vi "Joystick and Camera.vi"() -> ()   [LabVIEW 2021]
uses:
  Classes/Controller/Camera/Machine Vision.ctl
  Classes/Controller/Camera/Image processing.ctl
  Classes/Controller/Camera/Camera settings.ctl
  <vilib>/vision/Pattern Matching.llb/IMAQ GM Match Report.ctl
  <vilib>/vision/Measure.llb/Edge New.ctl
  Classes/Controller/I-O/I-O.lvclass
  Classes/Controller/Camera/Camera.lvclass
  Classes/Controller/Controller.lvclass
  Classes/Controller/Motion/A3200/A3200.lvclass
  Classes/Controller/Motion/Motion.lvclass
  Test VIs/Test VIs.lvclass
panel:
  in  "Cluster":T1={"Bayer"={"Algorithm"=0, "Gain R"=1.0, "Gain B"=1.0, "Gain G"=1.0, "Pattern"=5}, "Acquisition Control"={"Trigger Selector"=0, "Acquisition Frame Rate"=20.0, "Exposure Time"=100.0, "Acquisition Frame Rate Target"=20.0}, "Analog Control"={"Black Level"=0.0, "Gain Selector"=10, "Gain"=1.0}} {"Analog Control"."Gain" min=1.0 max=15.0; "Analog Control"."Gain Selector" items=["Analog All"=10, "Digital All"=20]; "Analog Control"."Black Level" min=0.0 max=255.9375; "Acquisition Control"."Acquisition Frame Rate Target" min=0.001 max=150000000.0; "Acquisition Control"."Exposure Time" min=27.793333333333333 max=1048539.7933333333; "Acquisition Control"."Acquisition Frame Rate" min=0.9536888685435264 max=30.757874015748033; "Acquisition Control"."Trigger Selector" items=["Frame Start"=3, "Exposure Start"=10]; "Bayer"."Pattern" items=["Use hardware value"=5, "None"=0, "GB"=1, "GR"=2, "BG"=3, "RG"=4]; "Bayer"."Gain G" min=0.0 max=3.999; "Bayer"."Gain B" min=0.0 max=3.999; "Bayer"."Gain R" min=0.0 max=3.999; "Bayer"."Algorithm" items=["Bilinear", "VNG"]}
  out "Used Edges (Adv. Straight Edge 1)":cluster{"Edge Information":T2[]}[](array[cluster]) {"Edge Information"."Distance (Real-World)" format="%.2f"; "Edge Information"."Location (Real-World)"."Y" format="%.2g"; "Edge Information"."Location (Real-World)"."X" format="%.2f"; "Edge Information"."Noise" format="%.2f"; "Edge Information"."Location (Pixel)"."Y" format="%.2g"; "Edge Information"."Location (Pixel)"."X" format="%.2f"; "Edge Information"."Strength" format="%.2f"; "Edge Information"."Distance (Pixel)" format="%.2f"}
  out "pattern matching":T3 {"Correlation Score" format="%.2f"; "Target Template Curve Score" format="%.2f"; "Template Target Curve Score" format="%.2f"; "Bounding Box"."y" format="%.2f"; "Bounding Box"."x" format="%.2f"; "Position"."y" format="%.2f"; "Position"."x" format="%.2f"; "Score" format="%.2f"; "Scale" format="%.2f"; "Angle" format="%.2f"; "Occlusion %" format="%.2f"}
  out "Match?":bool
  out "Current position spiral":dbl[](array[numeric])
  in  "Z high":dbl=12.5
  in  "XY high":dbl=50.0
  in  "Z low":dbl=0.05
  in  "XY low":dbl=0.1
  out "Current Z High Speed":dbl
  out "Current XY High Speed":dbl
  out "current Z low speed":dbl
  out "current XY speed":dbl
  out "High Speed":bool
  out "Z":bool
  out "Y":bool
  out "X":bool
  out "Low Speed":bool
  out "Global Report":T4 {"Mean Value" format="%.2f"; "%" format="%.2f"; "Area (calibrated)" format="%.2f"; "Maximal Value" format="%.2f"; "Minimal Value" format="%.2f"; "Standard Variation" format="%.2f"}
  in  "MoveFour":dbl[][](array[numeric])=[[1280.0, 960.0], [-2560.0, 0.0], [0.0, -1920.0], [2560.0, 0.0], [-1280.0, 960.0]]
  in  "Check four images":bool
  in  "Go TL fid":bool
  in  "Find fiducial":bool
  in  "Loop count":dbl=1.0
  in  "X, Y pixel stride":dbl[](array[numeric])=[1520.0, 2160.0]
  in  "Draw spiral":bool
  out "Move by":dbl[](array[numeric])
  in  "Find in Image":bool
  in  "Screen Grab":bool
  in  "Focus step size":dbl format="%#_13g"
  in  "number of focus steps":i32
  out "Radius (Real-World)":dbl
  out "error out":errorcluster
  in  "Find fiducial center":bool
  out "maximum is best focus":dbl
  in  "Focus":bool
  in  "Override presets":bool
  in  "Camera settings":T5={"Gamma"=1.6, "Gain"=0, "Sharpness"=0, "Contrast"=0.0, "Exposure"=0.0078125} {"Exposure" min=0.000244140625 max=0.5 scale=0.0002..0.5; "Contrast" min=0.0 max=1.0 scale=0.0..1.0; "Sharpness" min=0 max=2 step=1 scale=0.0..2.0; "Gain" min=0 max=100 step=1 scale=0.0..100.0; "Gamma" min=0.01 max=10.0 scale=0.01..10.0}
  in  "Image processing":T6={"Brightness"=128.0, "Contrast"=45.0, "Gamma"=1.0471123} {"Brightness" scale=0.0..400.0; "Contrast" scale=0.0..90.0; "Gamma" scale=0.005..5.0}
  out "XYZTheta Out":dbl[](array[numeric])
  in  "Machine Vision":T7
  in  "Move 10cm Right":bool
  in  "Move 10cm Backward":bool
  in  "Move 10cm Forward":bool
  in  "Move 10cm Left":bool
  in  "Record Measurement":bool=TRUE
  in  "Dismount Silicon Tray":bool
  in  "Secure Silicon Tray":bool
  in  "Z Go":bool
  in  "Position":dbl
  in  "XYZTheta":dbl[](array[numeric])
  in  "Go":bool
  in  "Joystick":bool
  out "Sum":dbl[](array[numeric]) format="%#.6g"
  out "Gantry":dbl[](array[numeric]) format="%#.6g"
  in  "Stop":bool
  out "Image":T8(plugin-control)
  out "Camera":dbl[](array[numeric])
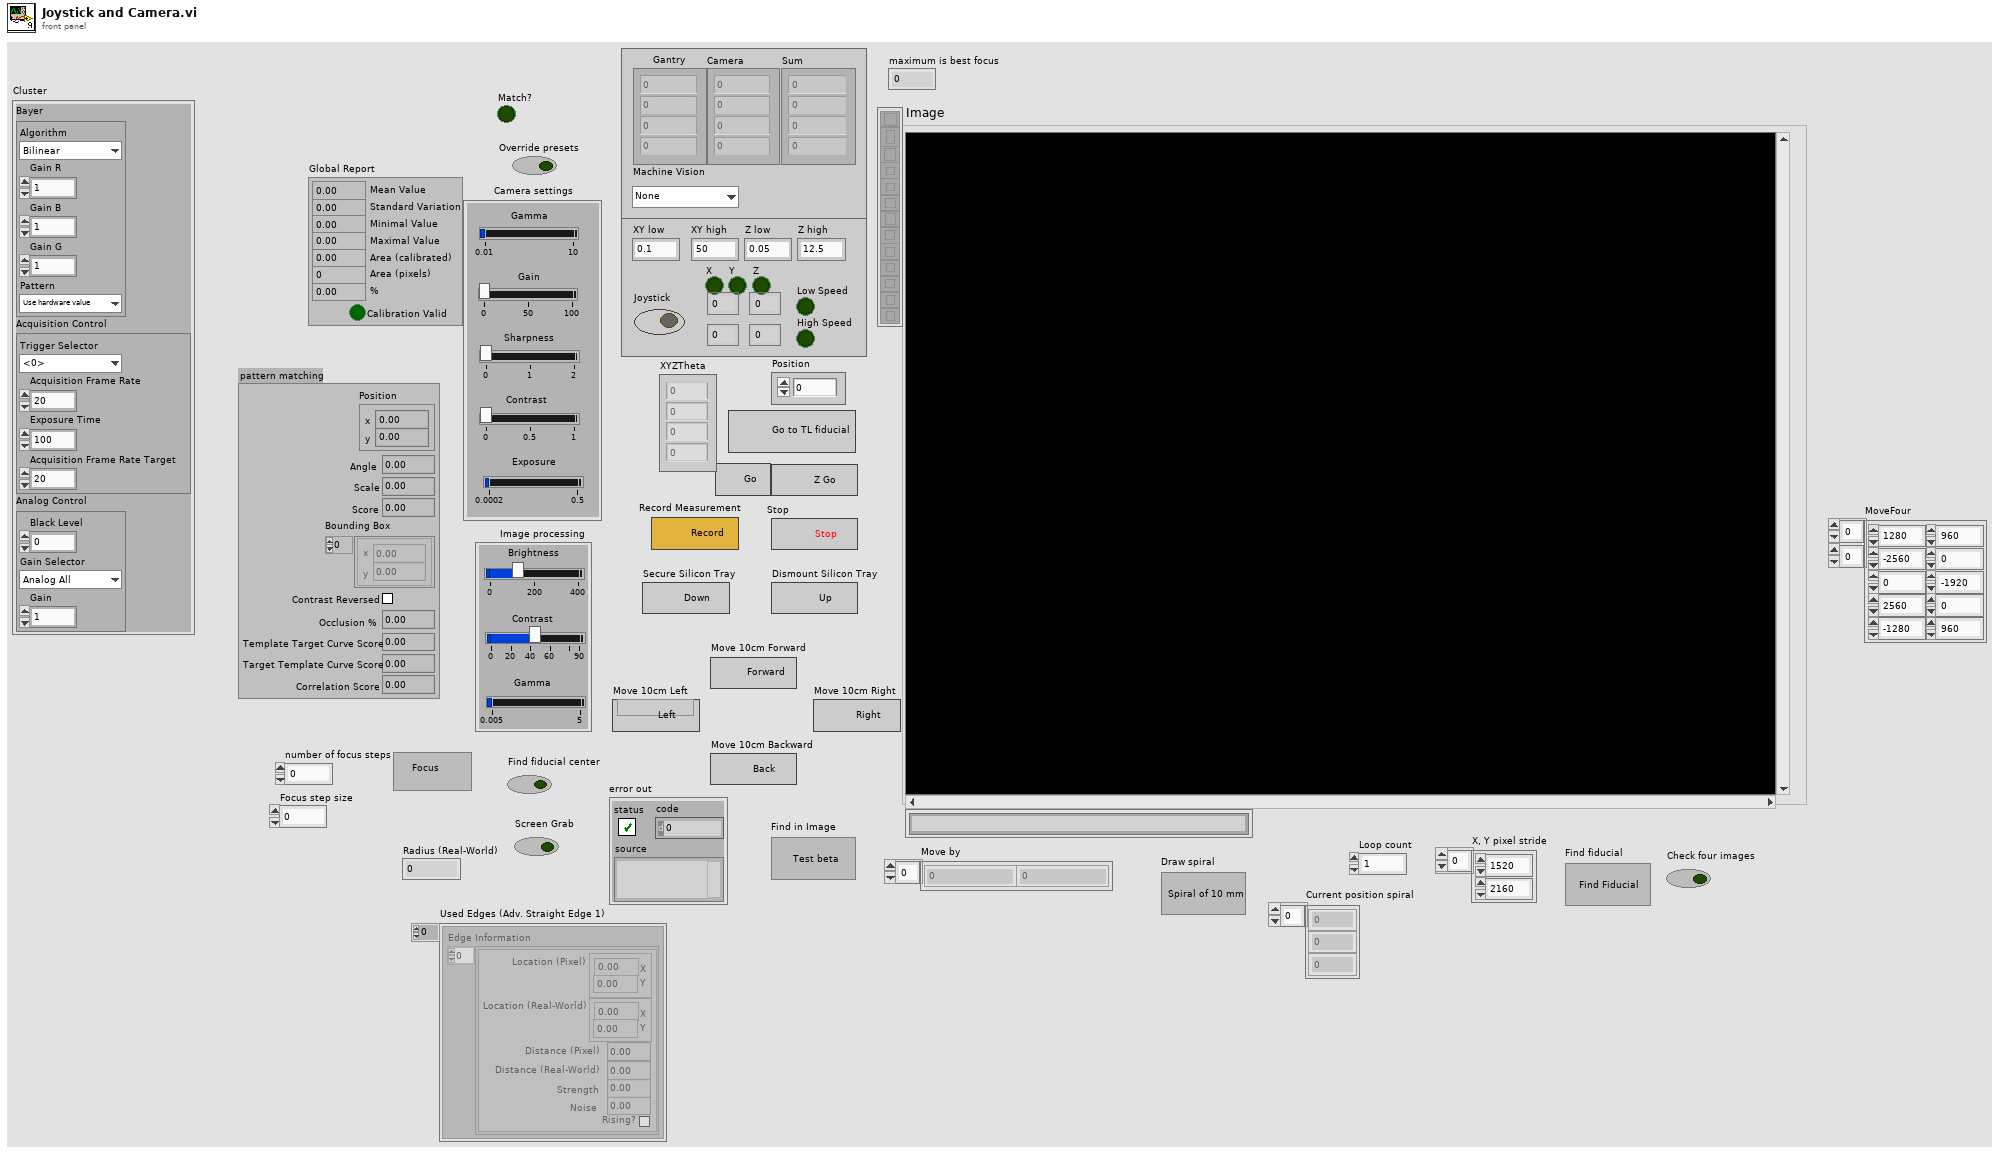
[diagram p1: front panel]
types:
  T1 = cluster{"Bayer":cluster{"Algorithm":u32, "Gain R":dbl, "Gain B":dbl, "Gain G":dbl, "Pattern":u32}, "Acquisition Control":cluster{"Trigger Selector":u32, "Acquisition Frame Rate":dbl, "Exposure Time":dbl, "Acquisition Frame Rate Target":dbl}, "Analog Control":cluster{"Black Level":dbl, "Gain Selector":u32, "Gain":dbl}}
  T2 = typedef "Edge New.ctl" = cluster{"Location (Pixel)":cluster{"X":sgl, "Y":sgl}, "Location (Real-World)":cluster{"X":sgl, "Y":sgl}, "Distance (Pixel)":dbl, "Distance (Real-World)":dbl, "Strength":dbl, "Noise":dbl, "Rising?":bool}
  T3 = typedef "IMAQ GM Match Report.ctl" = cluster{"Position":cluster{"x":sgl, "y":sgl}, "Angle":sgl, "Scale":sgl, "Score":sgl, "Bounding Box":cluster{"x":sgl, "y":sgl}[], "Contrast Reversed":bool, "Occlusion %":sgl, "Template Target Curve Score":sgl, "Target Template Curve Score":sgl, "Correlation Score":sgl}
  T4 = cluster{"Mean Value":sgl, "Standard Variation":sgl, "Minimal Value":sgl, "Maximal Value":sgl, "Area (calibrated)":sgl, "Area (pixels)":u32, "%":sgl, "Calibration Valid":bool}
  T5 = typedef "Camera.lvclass/Camera settings.ctl" = cluster{"Gamma":dbl, "Gain":i64, "Sharpness":i64, "Contrast":dbl, "Exposure":dbl}
  T6 = typedef "Camera.lvclass/Image processing.ctl" = cluster{"Brightness":sgl, "Contrast":sgl, "Gamma":sgl}
  T7 = typedef "Camera.lvclass/Machine Vision.ctl" = enum16{"None", "Assembly Tray Circle", "Assembly Tray Fiducial", "Partial Hexaboard", "sensor edge init", "HB edge init", "sensor edge pos1", "sensor edge pos2", "HB edge pos1", "HB edge pos2", "Sensor CH1-2", "HB CH1", "HB CH2", "V3 Sensor Circle", "Hexaboard Circle", "sensor CH1 check", "HB CH1 check ", "sensor ID"}
  T8 = typedef "IMAQ Image.ctl" = refnum<image>
  T9 = enum16{"open", "replace", "create", "open or create", "replace or create", "replace or create with confirmation"}
  T10 = typedef "Controller.lvclass/Controllers.ctl" = cluster{"I-O.lvclass":refnum<class "I-O.lvclass">, "Gantry":refnum<k24>, "Dispenser":refnum<visa-resource-name>}
  T11 = cluster{"Average Strength":dbl, "Radius (Real-World)":dbl, "Match found?":bool, "initial angle":sgl, "Global Report":cluster{"Mean Value":sgl, "Standard Variation":sgl, "Minimal Value":sgl, "Maximal Value":sgl, "Area (calibrated)":sgl, "Area (pixels)":u32, "%":sgl, "Calibration Valid":bool}}
  T12 = typedef "I-O.lvclass/Pin Map.ctl" = cluster{"Region Valves":i32[], "Extra Valves":dbl[][][], "Tool Primary Valve":i32, "Tool Secondary Valve":i32, "Region Sensors":i32[], "Extra Sensors":dbl[][][], "Tool Primary Sensor":dbl, "Tool Secondary Sensor":dbl, "Compression Sensor":dbl, "5V":i32, "Dispenser Sensor":dbl, "Light Curtain":i32}
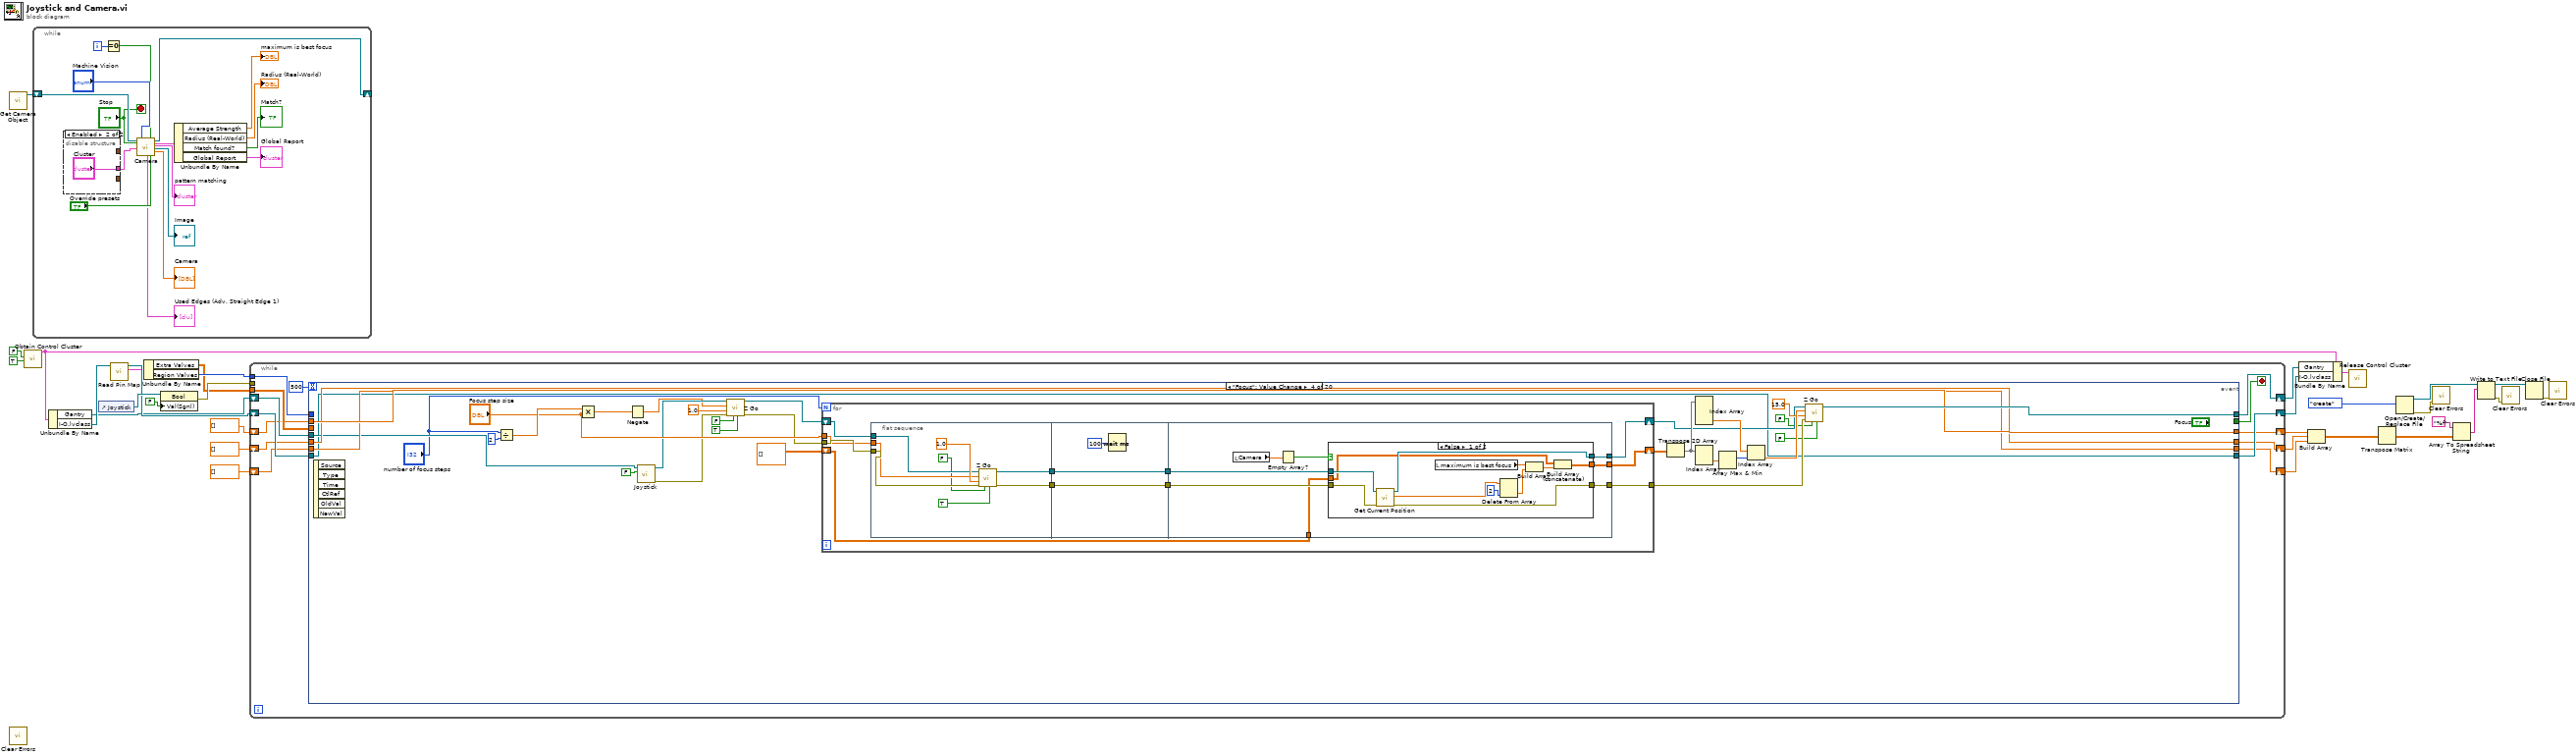
[diagram p0: block diagram]
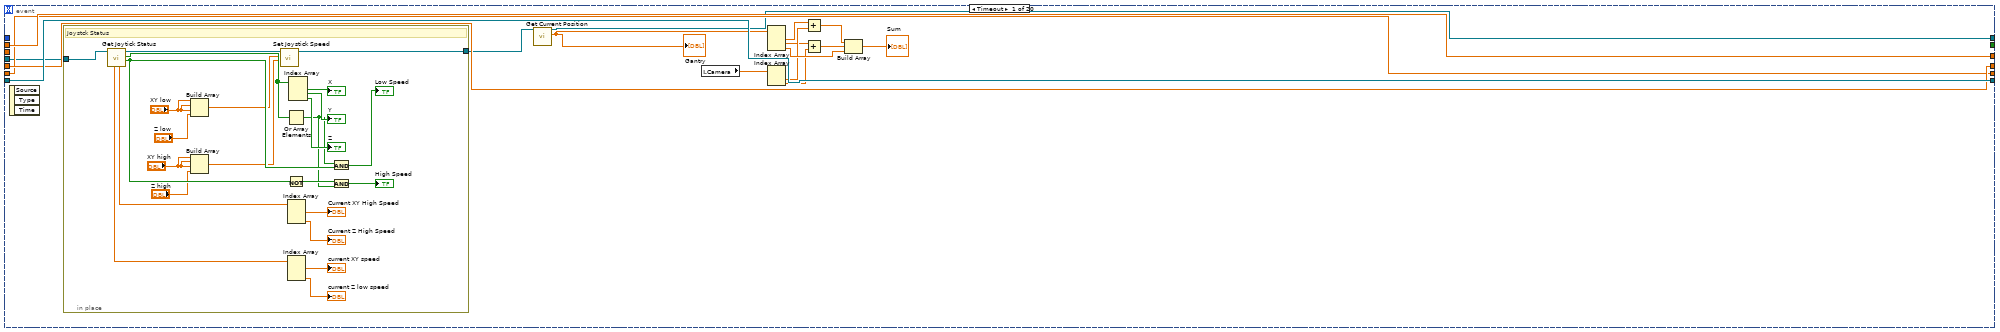
[diagram p2: hidden frame]
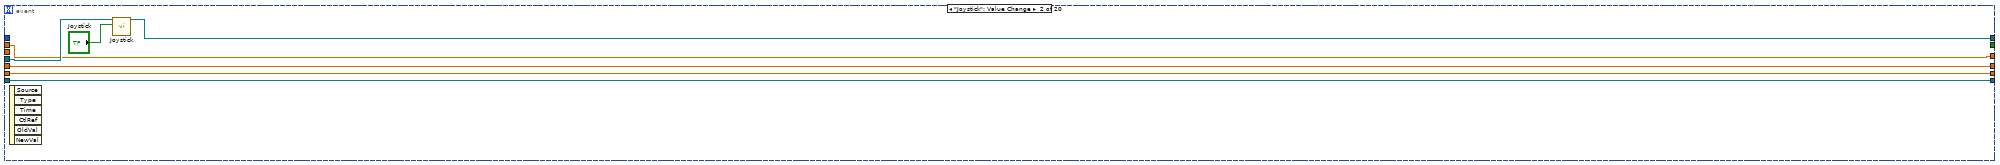
[diagram p3: hidden frame]
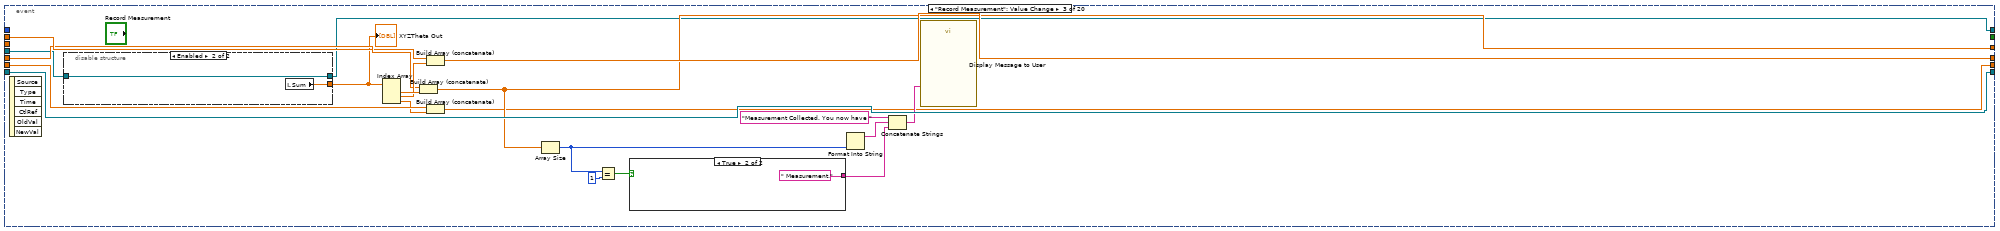
[diagram p4: hidden frame]
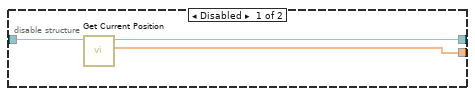
[diagram p5: hidden frame]
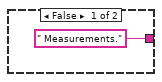
[diagram p6: hidden frame]
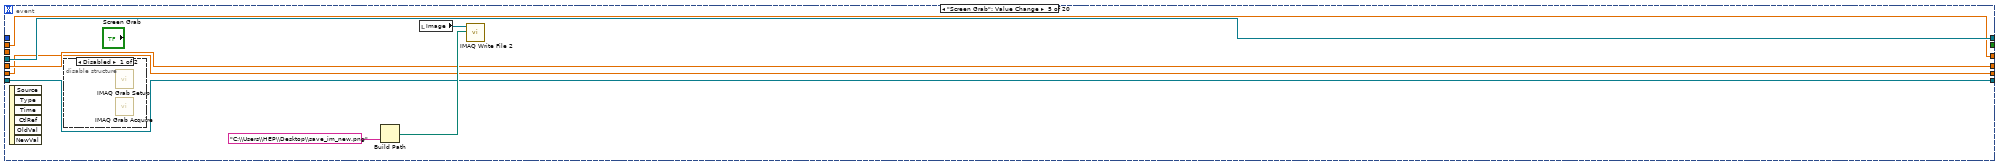
[diagram p8: hidden frame]
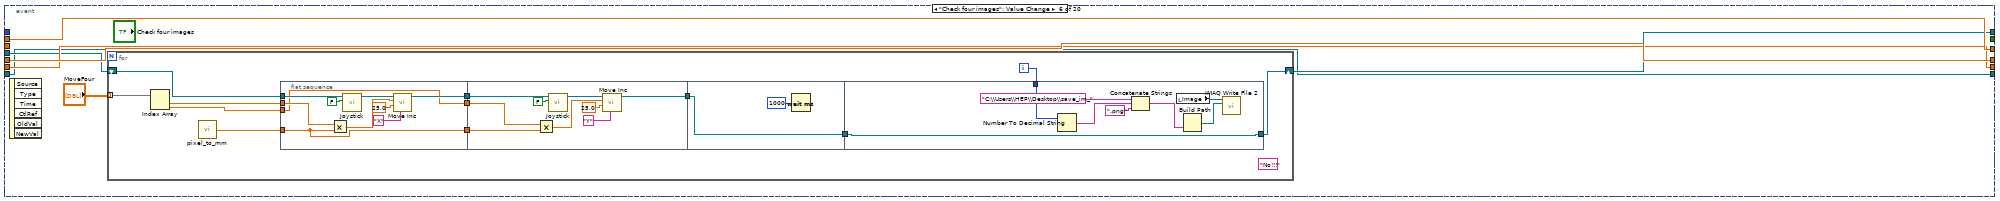
[diagram p10: hidden frame]
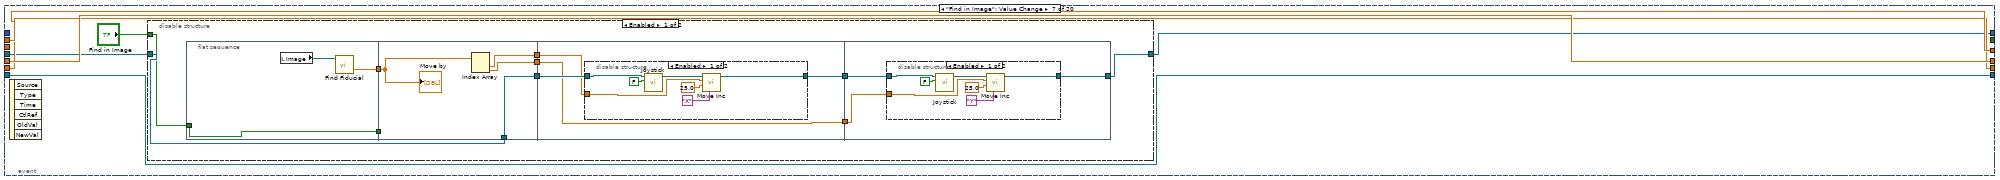
[diagram p11: hidden frame]
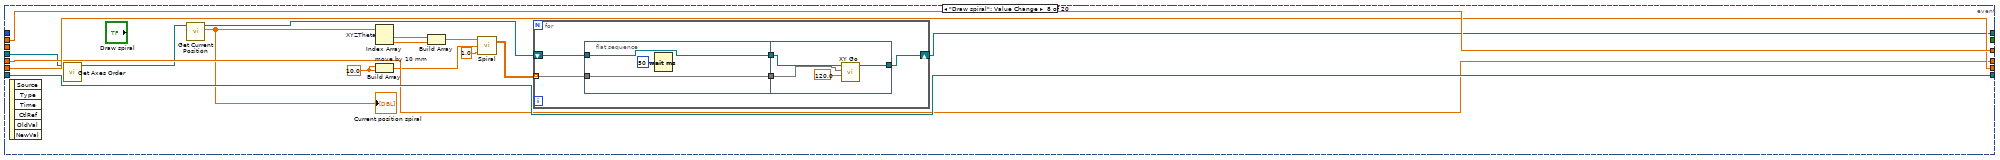
[diagram p15: hidden frame]
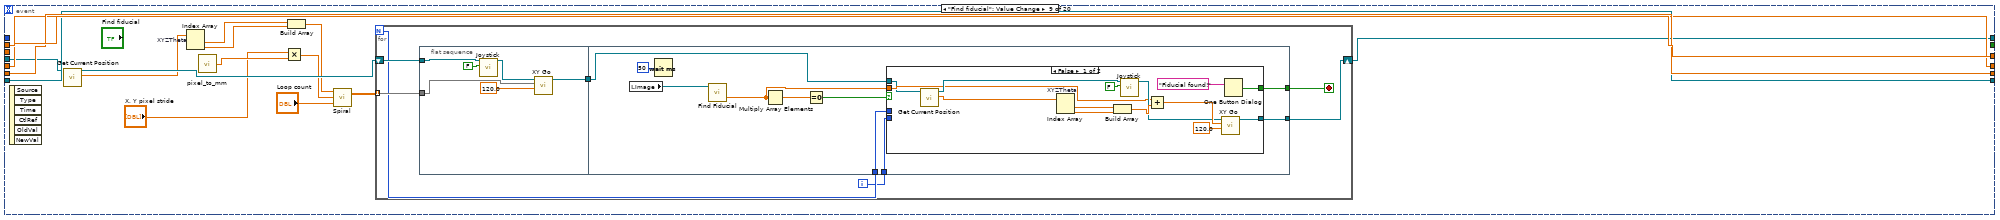
[diagram p16: hidden frame]
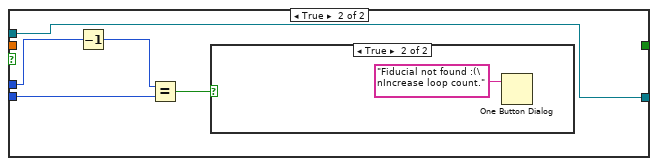
[diagram p17: hidden frame]
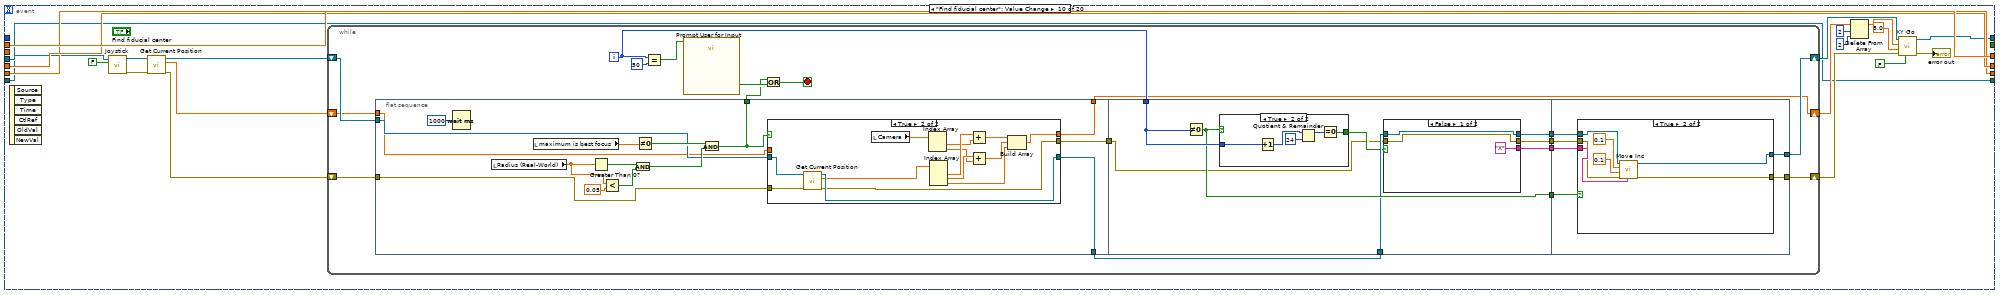
[diagram p19: hidden frame]
diagram:
  n1 = call "Get Camera Object.vi"() -> ("Camera out"=w27:refnum<class "Camera.lvclass">)  [unwired: 10 in, 1 out]
  n2 = call <vilib>:"Clear Errors.vi"() -> ()  [unwired: 6 in, 2 out]
  n3 = call "Obtain Control Cluster.vi"("I/O"=TRUE, "Dispense"=FALSE) -> ("Control Out"=w5:T10)  [unwired: 8 in, 1 out]
  n4 = while {
    shift-right: [w48] -> _
    shift-left: w27 -> [w49]
    i -> [w43]
    stop <- "Stop" stop-if-true
    n5 = disable-structure shown="Enabled" {
      disable-tunnel: ["Image processing" _] -> _
      disable-tunnel: ["Camera settings" _] -> _
      disable-tunnel: [_ "Cluster"] -> w33
      frame Disabled {
      }
      frame Enabled {
      }
    }
    n6 = Equal To 0?(x=w43) -> (x = 0?=w42:bool)
    n7 = call "Camera.vi"("Camera in"=w49, "Stop"="Stop", "Cluster"=w33, "Machine Vision"="Machine Vision", "Loop 0"=w42, "Override presets"="Override presets") -> ("Used Edges (Adv. Straight Edge 1)"=→"Used Edges (Adv. Straight Edge 1)":cluster{"Edge Information":T2[]}[], "Camera out"=w48:refnum<class "Camera.lvclass">, "output cluster"=w41:T11, "pattern matching"=→"pattern matching":T3, "Image"=→"Image":T8, "Camera"=→"Camera":dbl[])  [unwired: 6 in, 2 out]
    n8 = Unbundle By Name(w41) -> ("Average Strength"=→"maximum is best focus":dbl, "Radius (Real-World)"=→"Radius (Real-World)":dbl, "Match found?"=→"Match?":bool, "Global Report"=→"Global Report":T4)
  }
  n9 = Unbundle By Name(w5) -> ("Gantry"=w4:refnum<k24>, "I-O.lvclass"=w26:refnum<class "I-O.lvclass">)
  n10 = control-ref of="Joystick"() -> (w31:refnum<vi>)
  n11 = call-dynamic "Read Pin Map.vi"("I-O in"=w26) -> ("Pin Map 2"=w24:T12, "I-O out"=w25:refnum<class "I-O.lvclass">)  [unwired: 8 in, 1 out]
  n12 = Unbundle By Name(w24) -> ("Extra Valves"=w22:dbl[][][], "Region Valves"=w23:i32[])
  n13 = property class="Bool"(reference=w31, "Val(Sgnl)"=FALSE ("Value (Signaling)")) -> (error out=w30:errorcluster)  [unwired: 1 in, 1 out]
  n14 = while {
    shift-right: [w53] -> w8
    shift-left: w4 -> [w64]
    tunnel: w30 -> [_]
    shift-right: [w62] -> w7
    shift-left: w25 -> [w63]
    tunnel: w23 -> [w61]
    tunnel: w22 -> [w60]
    shift-right: [w55] -> w10
    shift-left: dbl[] [] -> [w59]
    shift-right: [w57] -> w11
    shift-left: dbl[] [] -> [w58]
    shift-right: [w54] -> w12
    shift-left: dbl[] [] -> [w56]
    stop <- w65 stop-if-true
    n15 = event shown="[3] \"Focus\": Value Change" {
      selector: _ -> [_ _ _ _ _ _ _ _ _ _ _ _ _ _ _ _ _ _ _ _]
      dyn-events: _ -> [_ _ _ _ _ _ _ _ _ _ _ _ _ _ _ _ _ _ _ _]
      timeout: 500 -> [_ _ _ _ _ _ _ _ _ _ _ _ _ _ _ _ _ _ _ _]
      tunnel: [_ _ _ _ _ _ _ _ _ _ _ _ _ _ _ _ _ _ _ TRUE] -> w65
      tunnel: w64 -> [w68 w114 w117 w159 w223 w229 w276 w323 w350 w426 w545 w556 w567 w578 w580 w590 w608 w627 w633 w670]
      tunnel: w63 -> [w83 w112 w134 w143 w222 w227 w280 w334 w363 w409 w540 w552 w564 w575 w587 w599 w605 w624 w637 w668]
      tunnel: [w83 w112 w134 w143 w222 w227 w280 w334 w363 w409 w540 w552 w564 w575 w584 w594 w605 w624 w637 w668] -> w62
      tunnel: w61 -> [_ _ _ _ _ _ _ _ _ _ _ _ _ _ w589 w598 _ _ _ _]
      tunnel: w60 -> [_ _ _ _ _ _ _ _ _ _ _ _ _ _ _ _ _ _ _ _]
      tunnel: w59 -> [w82 w111 w121 w162 w220 w231 w278 w333 w362 w428 w543 w555 w566 w577 w583 w593 w604 w623 w636 w667]
      tunnel: [w82 w111 w125 w162 w220 w231 w278 w333 w362 w428 w543 w555 w566 w577 w583 w593 w604 w623 w636 w667] -> w55
      tunnel: w58 -> [w81 w110 w122 w163 w221 w232 w279 w336 w365 w429 w542 w554 w565 w576 w582 w592 w603 w622 w635 w666]
      tunnel: [w81 w110 w124 w163 w221 w232 w279 w336 w365 w429 w542 w554 w565 w576 w582 w592 w603 w622 w635 w666] -> w57
      tunnel: w56 -> [w80 w109 w120 w161 w219 w230 w277 w335 w364 w427 w541 w553 w563 w574 w581 w591 w602 w621 w634 w665]
      tunnel: [w80 w109 w118 w161 w219 w230 w277 w335 w364 w427 w541 w553 w563 w574 w581 w591 w602 w621 w634 w665] -> w54
      tunnel: [w79 w108 w115 w164 w223 w228 w275 w332 w361 w423 w539 w548 w558 w570 w580 w590 w601 w620 w632 w663] -> w53
      event Timeout {
        n16 = event-data() -> ()  [unwired: 1 in, 3 out]
        n17 = in-place {
          in-place-border: w68 -> [w107]
          in-place-border: [w90] -> w67
          # "Joystck Status"
          n18 = call "Get Joytick Status.vi"("Gantry In"=w107) -> ("JoystickLowSpeedActive"=w101:bool, "Joystick Status"=w103:bool[], "Gantry Out"=w91:refnum<k24>, "High Speeds"=w94:dbl[], "Low Speeds"=w97:dbl[])  [unwired: 5 in, 1 out]
          n19 = Build Array("XY low", "XY low", "XY low", "Z low") -> (w87:dbl[])
          n20 = Build Array("XY high", "XY high", "XY high", "Z high") -> (w84:dbl[])
          n21 = call "Set Joystick Speed.vi"("High Speed Inputs"=w84, "Low Speed Inputs"=w87, "Gantry"=w91) -> ("Controller Out"=w90:refnum<k24>)  [unwired: 7 in, 1 out]
          n22 = Or Array Elements(Boolean array=w103) -> (logical OR=w99:bool)
          n23 = Not(x=w101) -> (.not. x?=w100:bool)
          n24 = Index Array(array=w94) -> (element #1=→"Current XY High Speed":dbl, element #3=→"Current Z High Speed":dbl)  [unwired: 3 in, 1 out]
          n25 = Index Array(array=w97) -> (element #1=→"current XY speed":dbl, element #3=→"current Z low speed":dbl)  [unwired: 3 in, 1 out]
          n26 = Index Array(array=w103) -> (element #1=→"X":bool, element #2=→"Y":bool, element #3=→"Z":bool)  [unwired: 3 in]
          n27 = And(x=w99, y=w101) -> (x .and. y?=→"Low Speed":bool)
          n28 = And(x=w100, y=w99) -> (x .and. y?=→"High Speed":bool)
        }
        n29 = call "Get Current Position.vi"("Gantry In"=w67) -> ("XYZTheta Out"=w76:dbl[], "Gantry Out"=w79:refnum<k24>)  [unwired: 8 in, 1 out]
        "Gantry" <- w76
        n30 = local read "Camera"() -> (w73:dbl[])
        n31 = Index Array(array=w76) -> (element #1=w74:dbl, element #2=w70:dbl, element #3=w77:dbl)  [unwired: 3 in]
        n32 = Index Array(array=w73) -> (element #1=w72:dbl, element #2=w69:dbl)  [unwired: 2 in]
        n33 = Add(x=w74, y=w72) -> (x+y=w75:dbl)
        n34 = Add(x=w70, y=w69) -> (x+y=w71:dbl)
        n35 = Build Array(w75, w71, w77) -> (→"Sum":dbl[])
      }
      event "Joystick": Value Change {
        n36 = event-data() -> ()  [unwired: 1 in, 6 out]
        n37 = call "Joystick.vi"("Joystick"="Joystick", "Gantry In"=w114) -> ("Gantry Out"=w108:refnum<k24>)  [unwired: 8 in, 1 out]
      }
      event "Record Measurement": Value Change {
        n38 = event-data() -> ()  [unwired: 1 in, 6 out]
        n39 = disable-structure shown="Enabled" {
          disable-tunnel: [w136 w138] -> w116
          disable-tunnel: w117 -> [w137 w139]
          disable-tunnel: [w135 w139] -> w115
          frame Disabled {
            n40 = call "Get Current Position.vi"("Gantry In"=w137) -> ("XYZTheta Out"=w136:dbl[], "Gantry Out"=w135:refnum<k24>)  [unwired: 8 in, 1 out]
          }
          frame Enabled {
            n41 = local read "Sum"() -> (w138:dbl[])
          }
        }
        "XYZTheta Out" <- w116
        n42 = Index Array(array=w116) -> (element #1=w133:dbl, element #2=w123:dbl, element #3=w119:dbl)  [unwired: 3 in]
        n43 = Build Array (concatenate) "Build Array"(w122, w133) -> (w124:dbl[])
        n44 = Build Array (concatenate)(w121, w123) -> (w125:dbl[])
        n45 = Build Array (concatenate)(w120, w119) -> (w118:dbl[])
        n46 = Array Size(array=w124) -> (size(s)=w128:i32)
        n47 = Equal?(x=w128, y=1) -> (x = y?=w127:bool)
        n48 = case shown="True" w127 {
          tunnel: [" Measurements." " Measurement."] -> w126
          frame False {
          }
          frame True {
          }
        }
        n49 = Format Into String(w128) -> (resulting string=w132:string)  [unwired: 3 in, 1 out]
        n50 = Concatenate Strings("Measurement Collected. You now have ", w132, w126) -> (w130:string)
        n51 = call "Display Message to User"("Message"=w130) -> ()  [unwired: 9 in, 2 out]
      }
      event "Focus": Value Change {
        n52 = event-data() -> ()  [unwired: 1 in, 6 out]
        n53 = Divide(x="number of focus steps", y=2) -> (x/y=w156:dbl)
        n54 = Multiply(x=w156, y="Focus step size") -> (x*y=w154:dbl)
        n55 = Negate(x=w154) -> (-x=w149:dbl)
        n56 = call "Joystick.vi"("Joystick"=FALSE, "Gantry In"=w159) -> ("error out"=w150:errorcluster, "Gantry Out"=w153:refnum<k24>)  [unwired: 8 in]
        n57 = call "Z Go.vi"("Increment"=TRUE, "Return Immediately"=FALSE ("Increment"), "error in (no error)"=w150, "Speed In"=1.0 ("Speed"), "Position In"=w149, "Gantry In"=w153) -> ("error out"=w151:errorcluster, "Gantry Out"=w152:refnum<k24>)  [unwired: 2 in, 2 out]
        n58 = for {
          N: "number of focus steps" -> [_]
          tunnel: w151 -> [w181]
          tunnel: [w180] -> w165
          shift-right: [w183] -> w166
          shift-left: w152 -> [w184]
          tunnel: "Focus step size" -> [w179]
          shift-right: [w182] -> w172
          shift-left: dbl[][] [] -> [w174]
          n59 = flat-sequence {
            tunnel: w184 -> [w191]
            tunnel: [w190] -> w178
            tunnel: w181 -> [w189]
            tunnel: [w188] -> w176
            tunnel: w179 -> [w187]
            tunnel: w178 -> [w195]
            tunnel: [w195] -> w177
            tunnel: w176 -> [w194]
            tunnel: [w194] -> w175
            tunnel: w177 -> [w199]
            tunnel: [w200] -> w183
            tunnel: [w197] -> w182
            tunnel: w175 -> [w198]
            tunnel: [w201] -> w180
            tunnel: w174 -> [w196]
            frame #0 {
              n60 = call "Z Go.vi"("Increment"=TRUE, "Return Immediately"=FALSE ("Increment"), "error in (no error)"=w189, "Speed In"=1.0 ("Speed"), "Position In"=w187, "Gantry In"=w191) -> ("error out"=w188:errorcluster, "Gantry Out"=w190:refnum<k24>)  [unwired: 2 in, 2 out]
            }
            frame #1 {
              n61 = Wait (ms)(milliseconds to wait=u32 100) -> ()  [unwired: 1 out]
            }
            frame #2 {
              n62 = local read "Camera"() -> (w203:dbl[])
              n63 = Empty Array?(array=w203) -> (empty?=w202:bool)
              n64 = case shown="False" w202 {
                tunnel: [w213 w215] -> w201
                tunnel: [w211 w216] -> w200
                tunnel: w199 -> [w210 w216]
                tunnel: w198 -> [w209 w215]
                tunnel: [w204 w217] -> w197
                tunnel: w196 -> [w206 w217]
                frame False {
                  n65 = call "Get Current Position.vi"("error in (no error)"=w209, "Gantry In"=w210) -> ("error out"=w213:errorcluster, "XYZTheta Out"=w212:dbl[], "Gantry Out"=w211:refnum<k24>)  [unwired: 7 in]
                  n66 = local read "maximum is best focus"() -> (w208:dbl)
                  n67 = Delete From Array(array=w212, index=2) -> (deleted portion=w207:dbl)  [unwired: 1 in, 1 out]
                  n68 = Build Array(w208, w207) -> (w205:dbl[])
                  n69 = Build Array (concatenate)(w206, w205) -> (w204:dbl[][])
                }
                frame True {
                }
              }
            }
          }
        }
        n70 = Transpose 2D Array(2D array=w172) -> (transposed array=w171:dbl[][])
        n71 = Index Array(array=w171) -> (element #2=w170:dbl[])  [unwired: 4 in, 1 out]
        n72 = Index Array(array=w171) -> (element=w173:dbl[])  [unwired: 2 in]
        n73 = Array Max & Min(array=w173) -> (max index (indices)=w169:i32)  [unwired: 3 out]
        n74 = Index Array(array=w170, index=w169) -> (element=w168:dbl)
        n75 = call "Z Go.vi"("Increment"=FALSE, "Return Immediately"=FALSE ("Increment"), "error in (no error)"=w165, "Speed In"=15.0 ("Speed"), "Position In"=w168, "Gantry In"=w166) -> ("Gantry Out"=w164:refnum<k24>)  [unwired: 2 in, 3 out]
      }
      event "Screen Grab": Value Change {
        n76 = event-data() -> ()  [unwired: 1 in, 6 out]
        n77 = disable-structure shown="Disabled" {
          frame Disabled {
            n78 = call <vilib>:"IMAQ Grab Setup.vi"() -> ()  [unwired: 10 in, 2 out]
            n79 = call <vilib>:"IMAQ Grab Acquire.vi"() -> ()  [unwired: 8 in, 4 out]
          }
          frame Enabled {
          }
        }
        n80 = Build Path(name or relative path="C:\\Users\\HEP\\Desktop\\save_im_new.png") -> (appended path=w225:path)  [unwired: 1 in]
        n81 = local read "Image"() -> (w218:T8)
        n82 = call-poly "IMAQ Write File 2"("File Path"=w225, "Image"=w218) -> ()  [unwired: 8 in, 2 out]
      }
      event "Check four images": Value Change {
        n83 = event-data() -> ()  [unwired: 1 in, 6 out]
        n84 = for {
          shift-right: [w242] -> w228
          shift-left: w229 -> [w243]
          tunnel: "MoveFour" -> [w241] mode=indexing
          i -> [w235]
          (unwired) "No!!!" ("F button name (\"Cancel\")")
          n85 = Index Array(array=w241) -> (element #1=w240:dbl, element #2=w238:dbl)  [unwired: 2 in]
          n86 = call "pixel_to_mm.vi"() -> ("mm/pixel"=w239:dbl)  [unwired: 2 in]
          n87 = flat-sequence {
            tunnel: [w250] -> w244
            tunnel: w243 -> [w249]
            tunnel: w240 -> [w248]
            tunnel: w239 -> [w245]
            tunnel: w238 -> [w246]
            tunnel: [w246] -> w237
            tunnel: [w245] -> w236
            tunnel: w244 -> [w259]
            tunnel: [w258] -> w234
            tunnel: w237 -> [w257]
            tunnel: w236 -> [w256]
            tunnel: w234 -> [w265]
            tunnel: [w265] -> w233
            tunnel: w233 -> [w271]
            tunnel: [w271] -> w242
            tunnel: w235 -> [w267]
            frame #0 {
              n88 = Multiply(x=w248, y=w245) -> (x*y=w247:dbl)
              n89 = call "Joystick.vi"("Joystick"=FALSE, "Gantry In"=w249) -> ("Gantry Out"=w251:refnum<k24>)  [unwired: 8 in, 1 out]
              n90 = call "Move Inc.vi"("Axis"="X", "Speed"=25.0, "Distance"=w247, "Gantry In"=w251) -> ("Gantry Out"=w250:refnum<k24>)  [unwired: 6 in, 1 out]
            }
            frame #1 {
              n91 = Multiply(x=w257, y=w256) -> (x*y=w255:dbl)
              n92 = call "Joystick.vi"("Joystick"=FALSE, "Gantry In"=w259) -> ("Gantry Out"=w260:refnum<k24>)  [unwired: 8 in, 1 out]
              n93 = call "Move Inc.vi"("Axis"="Y", "Speed"=25.0, "Distance"=w255, "Gantry In"=w260) -> ("Gantry Out"=w258:refnum<k24>)  [unwired: 6 in, 1 out]
            }
            frame #2 {
              n94 = Wait (ms)(milliseconds to wait=u32 1000) -> ()  [unwired: 1 out]
            }
            frame #3 {
              n95 = Number To Decimal String(number=w267) -> (decimal integer string=w266:string)  [unwired: 1 in]
              n96 = Concatenate Strings("C:\\Users\\HEP\\Desktop\\save_im_", w266, ".png") -> (w270:string)
              n97 = local read "Image"() -> (w273:T8)
              n98 = Build Path(name or relative path=w270) -> (appended path=w272:path)  [unwired: 1 in]
              n99 = call-poly "IMAQ Write File 2"("File Path"=w272, "Image"=w273) -> ()  [unwired: 8 in, 2 out]
            }
          }
        }
      }
      event "Find in Image": Value Change {
        n100 = event-data() -> ()  [unwired: 1 in, 6 out]
        n101 = disable-structure shown="Enabled" {
          disable-tunnel: w276 -> [w284 w321]
          disable-tunnel: [w283 w321] -> w275
          disable-tunnel: "Find in Image" -> [w282 _]
          frame Enabled {
            n102 = flat-sequence {
              tunnel: [w293] -> w290
              tunnel: w282 -> [w293]
              tunnel: [w292] -> w281
              tunnel: w290 -> [_]
              tunnel: w284 -> [w297]
              tunnel: [w297] -> w289
              tunnel: [w296] -> w288
              tunnel: [w295] -> w287
              tunnel: w281 -> [w294]
              tunnel: w289 -> [w301]
              tunnel: [w300] -> w286
              tunnel: w288 -> [w299]
              tunnel: [w298] -> w285
              tunnel: w287 -> [w298]
              tunnel: [w311] -> w283
              tunnel: w286 -> [w312]
              tunnel: w285 -> [w310]
              frame #0 {
                n103 = local read "Image"() -> (w291:T8)
                n104 = call "Find Fiducial.vi"("Image"=w291) -> ("Move by (mm)"=w292:dbl[])  [unwired: 3 in]
              }
              frame #1 {
                n105 = Index Array(array=w294) -> (element #1=w296:dbl, element #2=w295:dbl)  [unwired: 2 in]
                "Move by" <- w294
              }
              frame #2 {
                n106 = disable-structure shown="Enabled" {
                  disable-tunnel: w301 -> [w308 w309]
                  disable-tunnel: [w307 w309] -> w300
                  disable-tunnel: w299 -> [w306 _]
                  frame Enabled {
                    n107 = call "Joystick.vi"("Joystick"=FALSE, "Gantry In"=w308) -> ("Gantry Out"=w302:refnum<k24>)  [unwired: 8 in, 1 out]
                    n108 = call "Move Inc.vi"("Axis"="X", "Speed"=25.0, "Distance"=w306, "Gantry In"=w302) -> ("Gantry Out"=w307:refnum<k24>)  [unwired: 6 in, 1 out]
                  }
                  frame Disabled {
                  }
                }
              }
              frame #3 {
                n109 = disable-structure shown="Enabled" {
                  disable-tunnel: w312 -> [w319 w320]
                  disable-tunnel: [w318 w320] -> w311
                  disable-tunnel: w310 -> [w317 _]
                  frame Enabled {
                    n110 = call "Joystick.vi"("Joystick"=FALSE, "Gantry In"=w319) -> ("Gantry Out"=w313:refnum<k24>)  [unwired: 8 in, 1 out]
                    n111 = call "Move Inc.vi"("Axis"="Y", "Speed"=25.0, "Distance"=w317, "Gantry In"=w313) -> ("Gantry Out"=w318:refnum<k24>)  [unwired: 6 in, 1 out]
                  }
                  frame Disabled {
                  }
                }
              }
            }
          }
          frame Disabled {
          }
        }
      }
      event "Draw spiral": Value Change {
        w326 = 10.0 ("element")
        n112 = event-data() -> ()  [unwired: 1 in, 6 out]
        n113 = call "Get Axes Order.vi"("Gantry In"=w323) -> ("Gantry Out"=w322:refnum<k24>)  [unwired: 8 in, 2 out]
        n114 = call "Get Current Position.vi"("Gantry In"=w322) -> ("XYZTheta Out"=w324:dbl[], "Gantry Out"=w331:refnum<k24>)  [unwired: 8 in, 1 out]
        "Current position spiral" <- w324
        n115 = Index Array "XYZTheta"(array=w324) -> (element #1=w330:dbl, element #2=w329:dbl)  [unwired: 2 in]
        n116 = Build Array "move by 10 mm"(w326, w326) -> (w325:dbl[])
        n117 = Build Array(w330, w329) -> (w328:dbl[])
        n118 = call "Spiral.vi"("Loop count"=1.0, "X, Y stride (mm)"=w325, "XY center (mm)"=w328) -> ("Spiral coordinates"=w337:dbl[][])  [unwired: 1 in]
        n119 = for {
          tunnel: w337 -> [w342] mode=indexing
          shift-right: [w340] -> w332
          shift-left: w331 -> [w341]
          n120 = flat-sequence {
            tunnel: w341 -> [w344]
            tunnel: w342 -> [w345]
            tunnel: [w345] -> w339
            tunnel: [w344] -> w338
            tunnel: [w346] -> w340
            tunnel: w339 -> [w348]
            tunnel: w338 -> [w347]
            frame #0 {
              n121 = Wait (ms)(milliseconds to wait=u32 50) -> ()  [unwired: 1 out]
            }
            frame #1 {
              n122 = call "XY Go.vi"("Speed"=120.0, "XY In"=w348, "Gantry In"=w347) -> ("Gantry Out"=w346:refnum<k24>)  [unwired: 6 in, 2 out]
            }
          }
        }
      }
      event "Find fiducial": Value Change {
        n123 = event-data() -> ()  [unwired: 1 in, 6 out]
        n124 = call "Get Current Position.vi"("Gantry In"=w350) -> ("XYZTheta Out"=w359:dbl[], "Gantry Out"=w360:refnum<k24>)  [unwired: 8 in, 1 out]
        n125 = Index Array "XYZTheta"(array=w359) -> (element #1=w358:dbl, element #2=w357:dbl)  [unwired: 2 in]
        n126 = call "pixel_to_mm.vi"() -> ("mm/pixel"=w354:dbl)  [unwired: 2 in]
        n127 = Multiply(x="X, Y pixel stride", y=w354) -> (x*y=w353:dbl[])
        n128 = Build Array(w358, w357) -> (w356:dbl[])
        n129 = call "Spiral.vi"("Loop count"="Loop count", "X, Y stride (mm)"=w353, "XY center (mm)"=w356) -> ("Spiral coordinates"=w351:dbl[][])  [unwired: 1 in]
        n130 = for {
          N -> [w368]
          tunnel: w351 -> [w372] mode=indexing
          shift-right: [w370] -> w361
          shift-left: w360 -> [w371]
          i -> [w367]
          stop <- w369 stop-if-true
          n131 = flat-sequence {
            tunnel: [w373] -> w366
            tunnel: w371 -> [w375]
            tunnel: w372 -> [w374]
            tunnel: [w385] -> w370
            tunnel: [w387] -> w369
            tunnel: w368 -> [w384]
            tunnel: w367 -> [w383]
            tunnel: w366 -> [w382]
            frame #0 {
              n132 = call "Joystick.vi"("Joystick"=FALSE, "Gantry In"=w375) -> ("Gantry Out"=w378:refnum<k24>)  [unwired: 8 in, 1 out]
              n133 = call "XY Go.vi"("Speed"=120.0, "XY In"=w374, "Gantry In"=w378) -> ("Gantry Out"=w373:refnum<k24>)  [unwired: 6 in, 2 out]
            }
            frame #1 {
              n134 = local read "Image"() -> (w388:T8)
              n135 = Wait (ms)(milliseconds to wait=u32 50) -> ()  [unwired: 1 out]
              n136 = call "Find Fiducial.vi"("Image"=w388) -> ("Move by (mm)"=w386:dbl[])  [unwired: 3 in]
              n137 = Multiply Array Elements(1:w386) -> (0:w380:dbl)
              n138 = Equal To 0?(x=w380) -> (x = 0?=w379:bool)
              n139 = case shown="False" w379 {
                tunnel: [w392 _] -> w387
                tunnel: w386 -> [w391 _]
                tunnel: [w390 w403] -> w385
                tunnel: w384 -> [_ w405]
                tunnel: w383 -> [_ w404]
                tunnel: w382 -> [w389 w403]
                frame False {
                  n140 = call "Get Current Position.vi"("Gantry In"=w389) -> ("XYZTheta Out"=w397:dbl[], "Gantry Out"=w402:refnum<k24>)  [unwired: 8 in, 1 out]
                  n141 = Index Array "XYZTheta"(array=w397) -> (element #1=w398:dbl, element #2=w399:dbl)  [unwired: 2 in]
                  n142 = Build Array(w398, w399) -> (w400:dbl[])
                  n143 = call "Joystick.vi"("Joystick"=FALSE, "Gantry In"=w402) -> ("Gantry Out"=w396:refnum<k24>)  [unwired: 8 in, 1 out]
                  n144 = Add(x=w391, y=w400) -> (x+y=w401:dbl[])
                  n145 = call "XY Go.vi"("Speed"=120.0, "XY In"=w401, "Gantry In"=w396) -> ("Gantry Out"=w390:refnum<k24>)  [unwired: 6 in, 2 out]
                  n146 = One Button Dialog(message="Fiducial found!") -> (true=w392:bool)  [unwired: 1 in]
                }
                frame True {
                  n147 = Decrement(x=w405) -> (x-1=w407:i32)
                  n148 = Equal?(x=w407, y=w404) -> (x = y?=w406:bool)
                  n149 = case shown="True" w406 {
                    frame False {
                    }
                    frame True {
                      n150 = One Button Dialog(message="Fiducial not found :(\nIncrease loop count.") -> ()  [unwired: 1 in, 1 out]
                    }
                  }
                }
              }
            }
          }
        }
      }
      event "Find fiducial center": Value Change {
        n151 = event-data() -> ()  [unwired: 1 in, 6 out]
        n152 = call "Joystick.vi"("Joystick"=FALSE, "Gantry In"=w426) -> ("error out"=w415:errorcluster, "Gantry Out"=w417:refnum<k24>)  [unwired: 8 in]
        n153 = call "Get Current Position.vi"("error in (no error)"=w415, "Gantry In"=w417) -> ("error out"=w414:errorcluster, "XYZTheta Out"=w412:dbl[], "Gantry Out"=w416:refnum<k24>)  [unwired: 7 in]
        n154 = while {
          shift-right: [w446] -> w424
          shift-left: w416 -> [w435]
          shift-right: [w447] -> w422
          shift-left: w414 -> [w432]
          shift-right: [w430] -> w411
          shift-left: w412 -> [w433]
          i -> [w441]
          stop <- w439 stop-if-true
          n155 = flat-sequence {
            tunnel: [w459] -> w436
            tunnel: [w458] -> w430
            tunnel: w435 -> [w457]
            tunnel: [w456] -> w434
            tunnel: w433 -> [w455]
            tunnel: w432 -> [w454]
            tunnel: [w453] -> w431
            tunnel: w441 -> [w487]
            tunnel: [w486] -> w445
            tunnel: [w485] -> w444
            tunnel: w434 -> [w484]
            tunnel: [w483] -> w443
            tunnel: [w482] -> w442
            tunnel: w431 -> [w480]
            tunnel: [w508] -> w446
            tunnel: [w509] -> w447
            tunnel: w445 -> [w510]
            tunnel: w444 -> [w507]
            tunnel: w443 -> [w506]
            tunnel: w442 -> [w505]
            frame #0 {
              n156 = Wait (ms)(milliseconds to wait=u32 1000) -> ()  [unwired: 1 out]
              n157 = local read "Radius (Real-World)"() -> (w449:dbl)
              n158 = local read "maximum is best focus"() -> (w462:dbl)
              n159 = Greater Than 0?(x=w449) -> (x > 0?=w451:bool)
              n160 = Less?(x=w449, y=0.05) -> (x < y?=w450:bool)
              n161 = And(x=w451, y=w450) -> (x .and. y?=w460:bool)
              n162 = Not Equal To 0?(x=w462) -> (x != 0?=w461:bool)
              n163 = And(x=w461, y=w460) -> (x .and. y?=w459:bool)
              n164 = case shown="True" w459 {
                tunnel: [w464 w468] -> w458
                tunnel: w457 -> [w465 w479]
                tunnel: [w465 w478] -> w456
                tunnel: w455 -> [w464 _]
                tunnel: w454 -> [w463 w467]
                tunnel: [w463 w466] -> w453
                frame False {
                }
                frame True {
                  n165 = call "Get Current Position.vi"("error in (no error)"=w467, "Gantry In"=w479) -> ("error out"=w466:errorcluster, "XYZTheta Out"=w477:dbl[], "Gantry Out"=w478:refnum<k24>)  [unwired: 7 in]
                  n166 = local read "Camera"() -> (w475:dbl[])
                  n167 = Index Array(array=w475) -> (element #1=w472:dbl, element #2=w471:dbl)  [unwired: 2 in]
                  n168 = Index Array(array=w477) -> (element #1=w476:dbl, element #2=w473:dbl, element #3=w474:dbl)  [unwired: 3 in]
                  n169 = Add(x=w476, y=w472) -> (x+y=w470:dbl)
                  n170 = Add(x=w473, y=w471) -> (x+y=w469:dbl)
                  n171 = Build Array(w470, w469, w474) -> (w468:dbl[])
                }
              }
            }
            frame #1 {
              n172 = Not Equal To 0?(x=w487) -> (x != 0?=w485:bool)
              n173 = case shown="True" w485 {
                selector: w485 -> [w488 _]
                tunnel: [w488 w492] -> w481
                tunnel: w487 -> [_ w490]
                frame False {
                }
                frame True {
                  n174 = Increment(x=w490) -> (x+1=w489:i32)
                  n175 = Quotient & Remainder(x=w489, y=24) -> (x-y*floor(x/y)=w491:i32)  [unwired: 1 out]
                  n176 = Equal To 0?(x=w491) -> (x = 0?=w492:bool)
                }
              }
              n177 = case shown="False" w481 {
                tunnel: ["X" ("Axis") "Y" ("Axis")] -> w486
                tunnel: w484 -> [w495 w503]
                tunnel: [w495 w502] -> w483
                tunnel: [w494 w498] -> w482
                tunnel: w480 -> [w494 w497]
                frame False {
                }
                frame True {
                  n178 = call "Move Inc.vi"("Axis"="X", "error in (no error)"=w497, "Speed"=1.0, "Distance"=-2.4, "Gantry In"=w503) -> ("error out"=w498:errorcluster, "Gantry Out"=w502:refnum<k24>)  [unwired: 5 in]
                }
              }
            }
            frame #2 {
              n179 = case shown="True" w507 {
                tunnel: w510 -> [_ w535]
                tunnel: w505 -> [w511 w534]
                tunnel: w506 -> [w514 w532]
                tunnel: [w512 w531] -> w509
                tunnel: [w513 w530] -> w508
                frame False {
                  n180 = disable-structure shown="Enabled" {
                    disable-tunnel: w514 -> [w526 w528]
                    disable-tunnel: [w524 w528] -> w513
                    disable-tunnel: [w523 w527] -> w512
                    disable-tunnel: w511 -> [w521 w527]
                    frame Enabled {
                      n181 = call "Move Inc.vi"("Axis"="X", "error in (no error)"=w521, "Speed"=1.0, "Distance"=-0.8, "Gantry In"=w526) -> ("error out"=w522:errorcluster, "Gantry Out"=w525:refnum<k24>)  [unwired: 5 in]
                      n182 = call "Move Inc.vi"("Axis"="Y", "error in (no error)"=w522, "Speed"=1.0, "Distance"=-1.0, "Gantry In"=w525) -> ("error out"=w523:errorcluster, "Gantry Out"=w524:refnum<k24>)  [unwired: 5 in]
                    }
                    frame Disabled {
                    }
                  }
                }
                frame True {
                  n183 = call "Move Inc.vi"("Axis"=w535, "error in (no error)"=w534, "Speed"=0.1, "Distance"=0.1, "Gantry In"=w532) -> ("error out"=w531:errorcluster, "Gantry Out"=w530:refnum<k24>)  [unwired: 5 in]
                }
              }
            }
          }
          n184 = Equal?(x=w441, y=50) -> (x = y?=w438:bool)
          n185 = call "Prompt User for Input"("Enable"=w438) -> ("OK"=w437:bool)  [unwired: 17 in, 1 out]
          n186 = Or(x=w436, y=w437) -> (x .or. y?=w439:bool)
        }
        n187 = Delete From Array(array=w411, length=2, index=2) -> (array with subset deleted=w419:dbl[])  [unwired: 1 out]
        n188 = call "XY Go.vi"("return immediately"=FALSE, "error in (no error)"=w422, "Speed"=5.0, "XY In"=w419, "Gantry In"=w424) -> ("error out"=→"error out":errorcluster, "Gantry Out"=w423:refnum<k24>)  [unwired: 4 in, 1 out]
      }
      event "Move 10cm Left": Value Change {
        n189 = event-data() -> ()  [unwired: 1 in, 6 out]
        n190 = call "Joystick.vi"("Joystick"=FALSE, "Gantry In"=w545) -> ("Gantry Out"=w536:refnum<k24>)  [unwired: 8 in, 1 out]
        n191 = call "Move Inc.vi"("Axis"="X", "Speed"=25.0, "Distance"=-100.0, "Gantry In"=w536) -> ("Gantry Out"=w539:refnum<k24>)  [unwired: 6 in, 1 out]
      }
      event "Move 10cm Backward": Value Change {
        n192 = event-data() -> ()  [unwired: 1 in, 6 out]
        n193 = call "Joystick.vi"("Joystick"=FALSE, "Gantry In"=w556) -> ("Gantry Out"=w547:refnum<k24>)  [unwired: 8 in, 1 out]
        n194 = call "Move Inc.vi"("Axis"="Y", "Speed"=25.0, "Distance"=100.0, "Gantry In"=w547) -> ("Gantry Out"=w548:refnum<k24>)  [unwired: 6 in, 1 out]
      }
      event "Move 10cm Forward": Value Change {
        n195 = event-data() -> ()  [unwired: 1 in, 6 out]
        n196 = call "Joystick.vi"("Joystick"=FALSE, "Gantry In"=w567) -> ("Gantry Out"=w559:refnum<k24>)  [unwired: 8 in, 1 out]
        n197 = call "Move Inc.vi"("Axis"="Y", "Speed"=25.0, "Distance"=-100.0, "Gantry In"=w559) -> ("Gantry Out"=w558:refnum<k24>)  [unwired: 6 in, 1 out]
      }
      event "Move 10cm Right": Value Change {
        n198 = event-data() -> ()  [unwired: 1 in, 6 out]
        n199 = call "Joystick.vi"("Joystick"=FALSE, "Gantry In"=w578) -> ("Gantry Out"=w569:refnum<k24>)  [unwired: 8 in, 1 out]
        n200 = call "Move Inc.vi"("Axis"="X", "Speed"=25.0, "Distance"=100.0, "Gantry In"=w569) -> ("Gantry Out"=w570:refnum<k24>)  [unwired: 6 in, 1 out]
      }
      event "Dismount Silicon Tray": Value Change {
        n201 = event-data() -> ()  [unwired: 1 in, 6 out]
        n202 = Index Array(array=w589, index=1) -> (element=w586:i32)
        n203 = call-dynamic "Digital Write 1 Channel.vi"("Value"=FALSE, "Channel"=w586, "I-O.lvclass"=w587) -> ("I-O.lvclass 2"=w584:refnum<class "I-O.lvclass">)  [unwired: 7 in, 1 out]
      }
      event "Secure Silicon Tray": Value Change {
        n204 = event-data() -> ()  [unwired: 1 in, 6 out]
        n205 = Index Array(array=w598, index=1) -> (element=w596:i32)
        n206 = call-dynamic "Digital Write 1 Channel.vi"("Value"=TRUE, "Channel"=w596, "I-O.lvclass"=w599) -> ("I-O.lvclass 2"=w594:refnum<class "I-O.lvclass">)  [unwired: 7 in, 1 out]
      }
      event "Go": Value Change {
        n207 = event-data() -> ()  [unwired: 1 in, 6 out]
        n208 = for {
          tunnel: "XYZTheta" -> [w615] mode=indexing
          tunnel: [w613] -> w607 mode=indexing
          shift-right: [w611] -> w606
          shift-left: w608 -> [w612]
          i -> [w617]
          n209 = Equal To 0?(x=w615) -> (x = 0?=w616:bool)
          n210 = call "Get Current Position.vi"("Gantry In"=w612) -> ("XYZTheta Out"=w610:dbl[], "Gantry Out"=w611:refnum<k24>)  [unwired: 8 in, 1 out]
          n211 = Index Array(array=w610, index=w617) -> (element=w614:dbl)
          n212 = Select(t=w614, s=w616, f=w615) -> (s? t:f=w613:dbl)
        }
        n213 = call "ClearXYZTheta Go.vi"("Speed"=300.0, "XYZTheta In"=w607, "Gantry In"=w606) -> ("Gantry Out"=w601:refnum<k24>)  [unwired: 6 in, 2 out]
      }
      event "Z Go": Value Change {
        n214 = event-data() -> ()  [unwired: 1 in, 6 out]
        n215 = call "Z Go.vi"("Increment"=FALSE, "Return Immediately"=FALSE ("Increment"), "Speed In"=15.0 ("Speed"), "Position In"="Position", "Gantry In"=w627) -> ("Gantry Out"=w620:refnum<k24>)  [unwired: 3 in, 3 out]
      }
      event "Go TL fid": Value Change {
        n216 = event-data() -> ()  [unwired: 1 in, 6 out]
        n217 = Two Button Dialog(message="Do you want to go to X = 778.56, Y = 710.58, Z = 86.257?", 1:"No!!!" ("F button name (\"Cancel\")"), 2:"Yes" ("T button name (\"OK\")")) -> (T button?=w628:bool)
        n218 = case shown="True" w628 {
          tunnel: w633 -> [w638 w640]
          tunnel: [w638 w639] -> w632
          frame False {
          }
          frame True {
            n219 = flat-sequence {
              tunnel: [w643] -> w642
              tunnel: w640 -> [w646]
              tunnel: w642 -> [w656]
              tunnel: [w655] -> w641
              tunnel: [w660] -> w639
              tunnel: w641 -> [w657]
              frame #0 {
                n220 = call "Joystick.vi"("Joystick"=FALSE, "Gantry In"=w646) -> ("Gantry Out"=w644:refnum<k24>)  [unwired: 8 in, 1 out]
                n221 = call "Z Go.vi"("Increment"=FALSE, "Return Immediately"=FALSE, "Speed In"=15.0 ("Speed"), "Position In"=0.0, "Gantry In"=w644) -> ("Gantry Out"=w643:refnum<k24>)  [unwired: 3 in, 3 out]
              }
              frame #1 {
                n222 = Build Array(778.56 ("element"), 710.58 ("element")) -> (w654:dbl[])
                n223 = call "XY Go.vi"("Speed"=120.0, "XY In"=w654, "Gantry In"=w656) -> ("Gantry Out"=w655:refnum<k24>)  [unwired: 6 in, 2 out]
              }
              frame #2 {
                n224 = call "Z Go.vi"("Increment"=FALSE, "Return Immediately"=FALSE, "Speed In"=15.0, "Position In"=86.257, "Gantry In"=w657) -> ("Gantry Out"=w660:refnum<k24>)  [unwired: 3 in, 3 out]
              }
            }
          }
        }
      }
      event "Stop": Value Change {
        n225 = event-data() -> ()  [unwired: 1 in, 5 out]
        n226 = call "Joystick.vi"("Joystick"=FALSE, "Gantry In"=w670) -> ("Gantry Out"=w663:refnum<k24>)  [unwired: 8 in, 1 out]
      }
    }
  }
  n227 = Bundle By Name(cluster=w5, "Gantry"=w8, "I-O.lvclass"=w7) -> (w6:T10)
  n228 = Build Array(w11, w10, w12) -> (w16:dbl[][])
  n229 = call "Release Control Cluster.vi"("output cluster"=w6) -> ()  [unwired: 11 in]
  n230 = Transpose Matrix(1:w16) -> (0:w15:dbl[][])
  n231 = Open/Create/Replace File(operation (0:open)=T9."create") -> (refnum out=w14:refnum<file>, error out=w3:errorcluster)  [unwired: 5 in, 1 out]
  n232 = call <vilib>:"Clear Errors.vi"("error in (no error)"=w3) -> ()  [unwired: 5 in, 2 out]
  n233 = Array To Spreadsheet String(array=w15, 3:"%f" ("format string")) -> (spreadsheet string=w18:string)  [unwired: 1 in]
  n234 = Write to Text File(file (use dialog)=w14, text=w18) -> (refnum out=w17:refnum<file>, error out=w2:errorcluster)  [unwired: 2 in, 1 out]
  n235 = call <vilib>:"Clear Errors.vi"("error in (no error)"=w2) -> ()  [unwired: 5 in, 2 out]
  n236 = Close File(refnum=w17) -> (error out=w1:errorcluster)  [unwired: 1 in, 1 out]
  n237 = call <vilib>:"Clear Errors.vi"("error in (no error)"=w1) -> ()  [unwired: 5 in, 2 out]
